vi "WildDrive_v4.vi"(8 "Defense Mode":bool, 9 "Enter Pivot":bool, 10 "Turn Joystick":dbl, 11 "Speed Joystick":dbl=-0.0) -> (0 "Right Side Power":dbl, 3 "Left Side Power":dbl)   [LabVIEW 2018]
uses:
  <vilib>/Analysis/1siggen.llb/Ramp Pattern by Samples.vi
  <vilib>/Analysis/NI_AALBase.lvlib
panel:
  in  "Debug Mode":bool
  in  "Debug Speed":dbl(slide) min=-1.0 max=1.0 scale=-1.0..1.0
  in  "Square Speed":bool=TRUE
  in  "Feed Forward Coeff":dbl(slide)=0.05 min=0.0 max=0.2 scale=0.0..0.2
  in  "Max Pivot Turn (defense)":dbl(slide)=0.05 min=0.0 max=1.0 scale=0.0..1.0
  in  "Max Pivot Turn (offense)":dbl(slide)=0.05 min=0.0 max=1.0 scale=0.0..1.0
  in  "Tune Arc Turn":dbl(slide)=1.2 min=0.9 max=2.0 scale=0.9..2.0
  in  "Speed Joystick Deadband":dbl(slide)=0.05 min=0.0 max=1.0 scale=0.0..1.0
  in  "Turn Behavior":bool=TRUE
  out "Left Side Power":cluster{"Y":dbl[], "X":dbl[]}(graph)={"Y"=[0.0, 0.010101010101010102, 0.020202020202020204, 0.030303030303030304, 0.04040404040404041, 0.05050505050505051, 0.06060606060606061, 0.07070707070707072, 0.08080808080808081, 0.09090909090909091, 0.10101010101010102, 0.11111111111111112, 0.12121212121212122, 0.13131313131313133, 0.14141414141414144, 0.15151515151515152, 0.16161616161616163, 0.17171717171717174, 0.18181818181818182, 0.19191919191919193, 0.20202020202020204, 0.21212121212121213, 0.22222222222222224, 0.23232323232323235, 0.24242424242424243, 0.25252525252525254, 0.26262626262626265, 0.27272727272727276, 0.2828282828282829, 0.29292929292929293, 0.30303030303030304, 0.31313131313131315, 0.32323232323232326, 0.33333333333333337, 0.3434343434343435, 0.3535353535353536, 0.36363636363636365, 0.37373737373737376, 0.38383838383838387, 0.393939393939394, 0.4040404040404041, 0.4141414141414142, 0.42424242424242425, 0.43434343434343436, 0.4444444444444445, 0.4545454545454546, 0.4646464646464647, 0.4747474747474748, 0.48484848484848486, 0.494949494949495, 0.5050505050505051, 0.5151515151515152, 0.5252525252525253, 0.5353535353535354, 0.5454545454545455, 0.5555555555555556, 0.5656565656565657, 0.5757575757575758, 0.5858585858585859, 0.595959595959596, 0.6060606060606061, 0.6161616161616162, 0.6262626262626263, 0.6363636363636365, 0.6464646464646465, 0.6565656565656566, 0.6666666666666667, 0.6767676767676768, 0.686868686868687, 0.696969696969697, 0.7070707070707072, 0.7171717171717172, 0.7272727272727273, 0.7373737373737375, 0.7474747474747475, 0.7575757575757577, 0.7676767676767677, 0.7777777777777778, 0.787878787878788, 0.797979797979798, 0.8080808080808082, 0.8181818181818182, 0.8282828282828284, 0.8383838383838385, 0.8484848484848485, 0.8585858585858587, 0.8686868686868687, 0.8787878787878789, 0.888888888888889, 0.8989898989898991, 0.9090909090909092, 0.9191919191919192, 0.9292929292929294, 0.9393939393939394, 0.9494949494949496, 0.9595959595959597, 0.9696969696969697, 0.9797979797979799, 0.98989898989899, 1.0], "X"=[0.0]}
  out "Right Side Power":cluster{"Y":dbl[], "X":dbl[]}(graph)={"Y"=[0.0, 0.010101010101010102, 0.020202020202020204, 0.030303030303030304, 0.04040404040404041, 0.05050505050505051, 0.06060606060606061, 0.07070707070707072, 0.08080808080808081, 0.09090909090909091, 0.10101010101010102, 0.11111111111111112, 0.12121212121212122, 0.13131313131313133, 0.14141414141414144, 0.15151515151515152, 0.16161616161616163, 0.17171717171717174, 0.18181818181818182, 0.19191919191919193, 0.20202020202020204, 0.21212121212121213, 0.22222222222222224, 0.23232323232323235, 0.24242424242424243, 0.25252525252525254, 0.26262626262626265, 0.27272727272727276, 0.2828282828282829, 0.29292929292929293, 0.30303030303030304, 0.31313131313131315, 0.32323232323232326, 0.33333333333333337, 0.3434343434343435, 0.3535353535353536, 0.36363636363636365, 0.37373737373737376, 0.38383838383838387, 0.393939393939394, 0.4040404040404041, 0.4141414141414142, 0.42424242424242425, 0.43434343434343436, 0.4444444444444445, 0.4545454545454546, 0.4646464646464647, 0.4747474747474748, 0.48484848484848486, 0.494949494949495, 0.5050505050505051, 0.5151515151515152, 0.5252525252525253, 0.5353535353535354, 0.5454545454545455, 0.5555555555555556, 0.5656565656565657, 0.5757575757575758, 0.5858585858585859, 0.595959595959596, 0.6060606060606061, 0.6161616161616162, 0.6262626262626263, 0.6363636363636365, 0.6464646464646465, 0.6565656565656566, 0.6666666666666667, 0.6767676767676768, 0.686868686868687, 0.696969696969697, 0.7070707070707072, 0.7171717171717172, 0.7272727272727273, 0.7373737373737375, 0.7474747474747475, 0.7575757575757577, 0.7676767676767677, 0.7777777777777778, 0.787878787878788, 0.797979797979798, 0.8080808080808082, 0.8181818181818182, 0.8282828282828284, 0.8383838383838385, 0.8484848484848485, 0.8585858585858587, 0.8686868686868687, 0.8787878787878789, 0.888888888888889, 0.8989898989898991, 0.9090909090909092, 0.9191919191919192, 0.9292929292929294, 0.9393939393939394, 0.9494949494949496, 0.9595959595959597, 0.9696969696969697, 0.9797979797979799, 0.98989898989899, 1.0], "X"=[0.0]}
  in  "Turn Joystick Deadband":dbl(slide)=0.05 min=0.0 max=1.0 scale=0.0..1.0
  out "Speed Joystick Mapping":cluster{"Y":dbl[], "X":dbl[]}(graph)={"Y"=[0.0, 0.010101010101010102, 0.020202020202020204, 0.030303030303030304, 0.04040404040404041, 0.05050505050505051, 0.06060606060606061, 0.07070707070707072, 0.08080808080808081, 0.09090909090909091, 0.10101010101010102, 0.11111111111111112, 0.12121212121212122, 0.13131313131313133, 0.14141414141414144, 0.15151515151515152, 0.16161616161616163, 0.17171717171717174, 0.18181818181818182, 0.19191919191919193, 0.20202020202020204, 0.21212121212121213, 0.22222222222222224, 0.23232323232323235, 0.24242424242424243, 0.25252525252525254, 0.26262626262626265, 0.27272727272727276, 0.2828282828282829, 0.29292929292929293, 0.30303030303030304, 0.31313131313131315, 0.32323232323232326, 0.33333333333333337, 0.3434343434343435, 0.3535353535353536, 0.36363636363636365, 0.37373737373737376, 0.38383838383838387, 0.393939393939394, 0.4040404040404041, 0.4141414141414142, 0.42424242424242425, 0.43434343434343436, 0.4444444444444445, 0.4545454545454546, 0.4646464646464647, 0.4747474747474748, 0.48484848484848486, 0.494949494949495, 0.5050505050505051, 0.5151515151515152, 0.5252525252525253, 0.5353535353535354, 0.5454545454545455, 0.5555555555555556, 0.5656565656565657, 0.5757575757575758, 0.5858585858585859, 0.595959595959596, 0.6060606060606061, 0.6161616161616162, 0.6262626262626263, 0.6363636363636365, 0.6464646464646465, 0.6565656565656566, 0.6666666666666667, 0.6767676767676768, 0.686868686868687, 0.696969696969697, 0.7070707070707072, 0.7171717171717172, 0.7272727272727273, 0.7373737373737375, 0.7474747474747475, 0.7575757575757577, 0.7676767676767677, 0.7777777777777778, 0.787878787878788, 0.797979797979798, 0.8080808080808082, 0.8181818181818182, 0.8282828282828284, 0.8383838383838385, 0.8484848484848485, 0.8585858585858587, 0.8686868686868687, 0.8787878787878789, 0.888888888888889, 0.8989898989898991, 0.9090909090909092, 0.9191919191919192, 0.9292929292929294, 0.9393939393939394, 0.9494949494949496, 0.9595959595959597, 0.9696969696969697, 0.9797979797979799, 0.98989898989899, 1.0], "X"=[0.0]}
  out "Turn Joystick Mapping":cluster{"Y":dbl[], "X":dbl[]}(graph)={"Y"=[0.0, 0.010101010101010102, 0.020202020202020204, 0.030303030303030304, 0.04040404040404041, 0.05050505050505051, 0.06060606060606061, 0.07070707070707072, 0.08080808080808081, 0.09090909090909091, 0.10101010101010102, 0.11111111111111112, 0.12121212121212122, 0.13131313131313133, 0.14141414141414144, 0.15151515151515152, 0.16161616161616163, 0.17171717171717174, 0.18181818181818182, 0.19191919191919193, 0.20202020202020204, 0.21212121212121213, 0.22222222222222224, 0.23232323232323235, 0.24242424242424243, 0.25252525252525254, 0.26262626262626265, 0.27272727272727276, 0.2828282828282829, 0.29292929292929293, 0.30303030303030304, 0.31313131313131315, 0.32323232323232326, 0.33333333333333337, 0.3434343434343435, 0.3535353535353536, 0.36363636363636365, 0.37373737373737376, 0.38383838383838387, 0.393939393939394, 0.4040404040404041, 0.4141414141414142, 0.42424242424242425, 0.43434343434343436, 0.4444444444444445, 0.4545454545454546, 0.4646464646464647, 0.4747474747474748, 0.48484848484848486, 0.494949494949495, 0.5050505050505051, 0.5151515151515152, 0.5252525252525253, 0.5353535353535354, 0.5454545454545455, 0.5555555555555556, 0.5656565656565657, 0.5757575757575758, 0.5858585858585859, 0.595959595959596, 0.6060606060606061, 0.6161616161616162, 0.6262626262626263, 0.6363636363636365, 0.6464646464646465, 0.6565656565656566, 0.6666666666666667, 0.6767676767676768, 0.686868686868687, 0.696969696969697, 0.7070707070707072, 0.7171717171717172, 0.7272727272727273, 0.7373737373737375, 0.7474747474747475, 0.7575757575757577, 0.7676767676767677, 0.7777777777777778, 0.787878787878788, 0.797979797979798, 0.8080808080808082, 0.8181818181818182, 0.8282828282828284, 0.8383838383838385, 0.8484848484848485, 0.8585858585858587, 0.8686868686868687, 0.8787878787878789, 0.888888888888889, 0.8989898989898991, 0.9090909090909092, 0.9191919191919192, 0.9292929292929294, 0.9393939393939394, 0.9494949494949496, 0.9595959595959597, 0.9696969696969697, 0.9797979797979799, 0.98989898989899, 1.0], "X"=[-0.0]}
  # "Driver Inputs"
  # "Tuning Parameters"
  # "Debug"
  # "Drive Outputs"
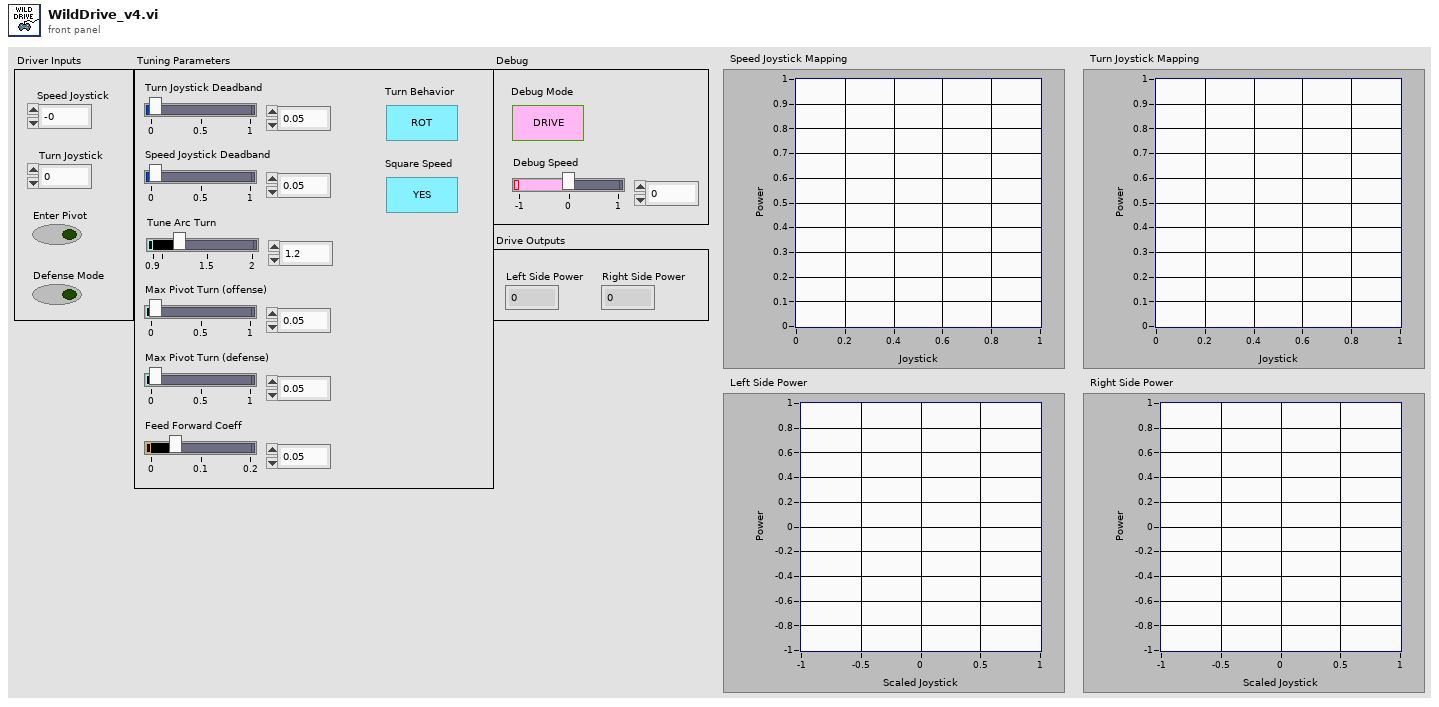
[diagram p1: front panel]
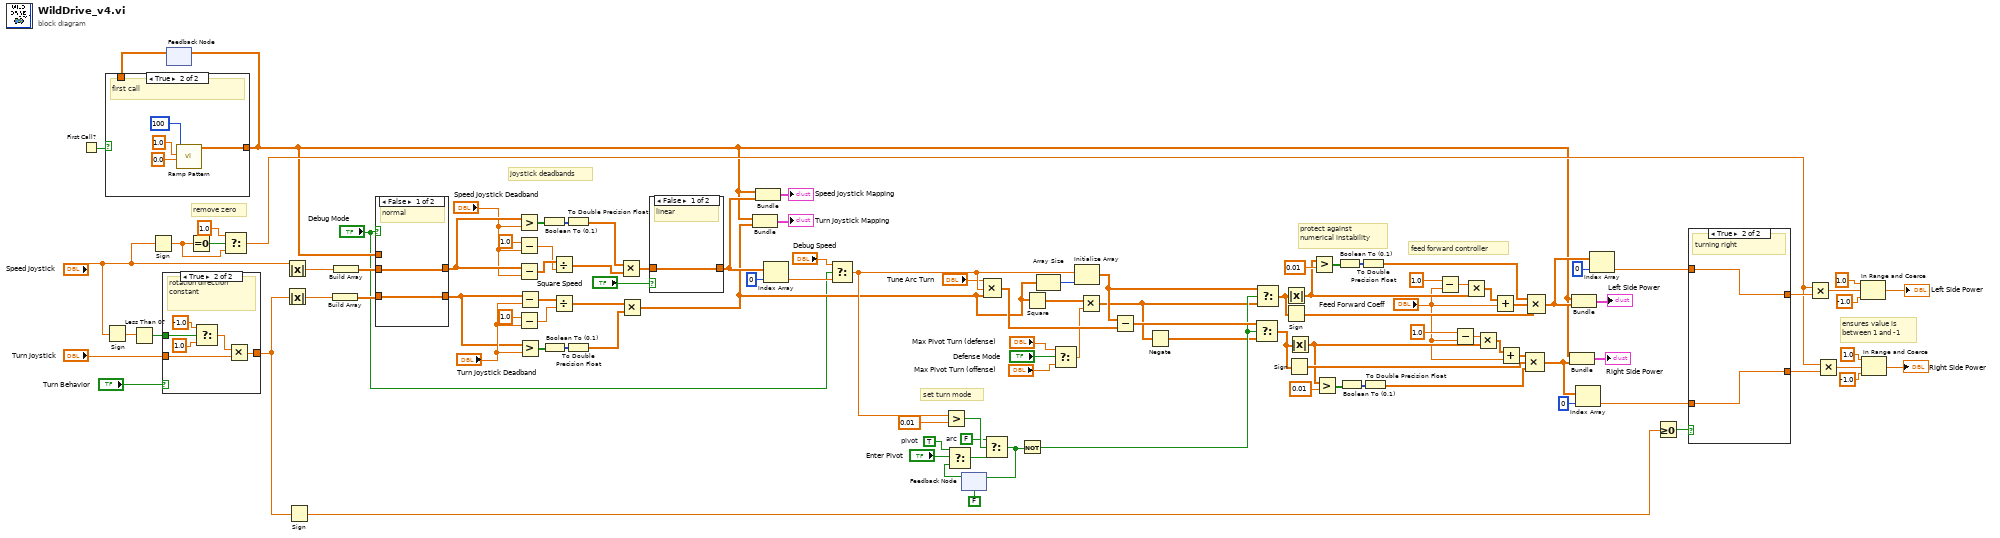
[diagram p0: block diagram]
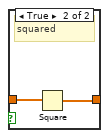
[diagram p6: hidden frame]
diagram:
  w12 = TRUE  # pivot
  w72 = FALSE  # arc
  # "remove zero"
  # "protect against\nnumerical instability"
  # "ensures value is \nbetween 1 and -1"
  # "set turn mode"
  # "feed forward controller"
  # "joystick deadbands"
  n1 = First Call?() -> (First Call?: T/F=w15:bool)
  n2 = Sign(1:"Speed Joystick") -> (0:w26:dbl)
  n3 = Less Than 0?(x=w26) -> (x < 0?=w27:bool)
  n4 = Sign(1:"Speed Joystick") -> (0:w19:dbl)
  n5 = case shown="True" "Turn Behavior" {
    tunnel: w27 -> [_ w117]
    tunnel: [w112 w114] -> w22
    tunnel: "Turn Joystick" -> [w112 w113]
    frame False {
      # "like a car"
    }
    frame True {
      # "rotation direction constant"
      n6 = Select(t=-1.0, s=w117, f=1.0) -> (s? t:f=w118:dbl)
      n7 = Multiply(x=w118, y=w113) -> (x*y=w114:dbl)
    }
  }
  n8 = feedback #1() -> (w13:dbl[])  [unwired: 1 in]
  n9 = case shown="True" w15 {
    tunnel: [w119 w120] -> w14
    tunnel: w13 -> [w119 _]
    frame False {
      # "subsequent calls"
    }
    frame True {
      # "first call"
      n10 = call-poly <vilib>:"Ramp Pattern.vi"("start"=0.0, "end"=1.0, "samples"=100) -> ("Ramp Pattern"=w120:dbl[])  [unwired: 7 in, 1 out]
    }
  }
  n11 = feedback-in #1(w14) -> ()
  n12 = Equal To 0?(x=w19) -> (x = 0?=w21:bool)
  n13 = Select(t=1.0, s=w21, f=w19) -> (s? t:f=w18:dbl)
  n14 = Absolute Value(x="Speed Joystick") -> (abs(x)=w108:dbl)
  n15 = Absolute Value(x=w22) -> (abs(x)=w111:dbl)
  n16 = Sign(1:w22) -> (0:w32:dbl)
  n17 = Build Array(w111) -> (w109:dbl[])
  n18 = Build Array(w108) -> (w110:dbl[])
  n19 = case shown="False" "Debug Mode" {
    tunnel: w14 -> [_ w126]
    tunnel: [w125 w126] -> w99
    tunnel: [w124 w126] -> w90
    tunnel: w110 -> [w125 _]
    tunnel: w109 -> [w124 _]
    frame False {
      # "normal"
    }
    frame True {
      # "debug"
    }
  }
  n20 = Greater?(x=w99, y="Speed Joystick Deadband") -> (0:w105:bool[])
  n21 = Subtract(x=1.0, y="Speed Joystick Deadband") -> (x-y=w96:dbl)
  n22 = Subtract(x=w99, y="Speed Joystick Deadband") -> (x-y=w98:dbl[])
  n23 = Subtract(x=1.0, y="Turn Joystick Deadband") -> (x-y=w92:dbl)
  n24 = Subtract(x=w90, y="Turn Joystick Deadband") -> (x-y=w94:dbl[])
  n25 = Greater?(x=w90, y="Turn Joystick Deadband") -> (0:w103:bool[])
  n26 = Boolean To (0,1)(Boolean=w105) -> (0, 1=w104:i16[])
  n27 = Boolean To (0,1)(Boolean=w103) -> (0, 1=w102:i16[])
  n28 = Divide(x=w98, y=w96) -> (x/y=w95:dbl[])
  n29 = Divide(x=w94, y=w92) -> (x/y=w89:dbl[])
  n30 = To Double Precision Float(number=w104) -> (double precision float=w101:dbl[])
  n31 = To Double Precision Float(number=w102) -> (double precision float=w88:dbl[])
  n32 = Multiply(x=w101, y=w95) -> (x*y=w100:dbl[])
  n33 = Multiply(x=w89, y=w88) -> (x*y=w3:dbl[])
  n34 = case shown="False" "Square Speed" {
    tunnel: w100 -> [w127 w129]
    tunnel: [w127 w128] -> w76
    frame False {
      # "linear"
    }
    frame True {
      # "squared"
      n35 = Square(x=w129) -> (x^2=w128:dbl[])
    }
  }
  n36 = Bundle("Ramp Pattern"=w14, w3) -> (→"Turn Joystick Mapping":cluster{"Ramp Pattern":dbl[], dbl[]})  [unwired: 1 in]
  n37 = Bundle("Ramp Pattern"=w14, w76) -> (→"Speed Joystick Mapping":cluster{"Ramp Pattern":dbl[], dbl[]})  [unwired: 1 in]
  n38 = Index Array(array=w76, index=0) -> (element=w78:dbl)
  n39 = Select(t="Debug Speed", s="Debug Mode", f=w78) -> (s? t:f=w31:dbl)
  n40 = Greater?(x=w31, y=0.01) -> (0:w74:bool)
  n41 = feedback #2(FALSE) -> (w80:bool)
  n42 = Select(t=w12, s="Enter Pivot", f=w80) -> (s? t:f=w73:bool)
  n43 = Compound Arithmetic op=MULTIPLY("Tune Arc Turn", w31, w3) -> (w82:dbl[])
  n44 = Select(t=w72, s=w74, f=w73) -> (s? t:f=w71:bool)
  n45 = feedback-in #2(w71) -> ()
  n46 = Not(x=w71) -> (.not. x?=w70:bool)
  n47 = Square(x=w3) -> (x^2=w17:dbl[])
  n48 = Array Size(array=w3) -> (size(s)=w87:i32)
  n49 = Select(t="Max Pivot Turn (defense)", s="Defense Mode", f="Max Pivot Turn (offense)") -> (s? t:f=w11:dbl)
  n50 = Initialize Array(w31, w87) -> (w86:dbl[])
  n51 = Multiply(x=w17, y=w11) -> (x*y=w16:dbl[])
  n52 = Subtract(x=w86, y=w82) -> (x-y=w85:dbl[])
  n53 = Negate(x=w16) -> (-x=w69:dbl[])
  n54 = Select(t=w85, s=w70, f=w69) -> (s? t:f=w30:dbl[])
  n55 = Select(t=w86, s=w70, f=w16) -> (s? t:f=w52:dbl[])
  n56 = Sign(1:w52) -> (0:w65:dbl[])
  n57 = Absolute Value(x=w52) -> (abs(x)=w28:dbl[])
  n58 = Sign(1:w30) -> (0:w60:dbl[])
  n59 = Absolute Value(x=w30) -> (abs(x)=w29:dbl[])
  n60 = Greater?(x=w28, y=0.01) -> (0:w55:bool[])
  n61 = Greater?(x=w29, y=0.01) -> (0:w59:bool[])
  n62 = Boolean To (0,1)(Boolean=w55) -> (0, 1=w54:i16[])
  n63 = Boolean To (0,1)(Boolean=w59) -> (0, 1=w58:i16[])
  n64 = To Double Precision Float(number=w54) -> (double precision float=w51:dbl[])
  n65 = To Double Precision Float(number=w58) -> (double precision float=w56:dbl[])
  n66 = Subtract(x=1.0, y="Feed Forward Coeff") -> (x-y=w67:dbl)
  n67 = Subtract(x=1.0, y="Feed Forward Coeff") -> (x-y=w63:dbl)
  n68 = Multiply(x=w67, y=w28) -> (x*y=w66:dbl[])
  n69 = Multiply(x=w63, y=w29) -> (x*y=w62:dbl[])
  n70 = Add(x=w66, y="Feed Forward Coeff") -> (x+y=w50:dbl[])
  n71 = Add(x=w62, y="Feed Forward Coeff") -> (x+y=w61:dbl[])
  n72 = Compound Arithmetic op=MULTIPLY(w61, w60, w56) -> (w48:dbl[])
  n73 = Compound Arithmetic op=MULTIPLY(w51, w50, w65) -> (w46:dbl[])
  n74 = Bundle("Ramp Pattern"=w14, w48) -> (→"Right Side Power":cluster{"Ramp Pattern":dbl[], dbl[]})  [unwired: 1 in]
  n75 = Bundle("Ramp Pattern"=w14, w46) -> (→"Left Side Power":cluster{"Ramp Pattern":dbl[], dbl[]})  [unwired: 1 in]
  n76 = Index Array(array=w48, index=0) -> (element=w35:dbl)
  n77 = Index Array(array=w46, index=0) -> (element=w37:dbl)
  n78 = Greater Or Equal To 0?(x=w32) -> (x >= 0?=w33:bool)
  n79 = case shown="True" w33 {
    tunnel: w37 -> [w131 w133]
    tunnel: [w130 w133] -> w36
    tunnel: w35 -> [w130 w132]
    tunnel: [w131 w132] -> w34
    frame False {
      # "turning left"
    }
    frame True {
      # "turning right"
    }
  }
  n80 = Multiply(x=w18, y=w36) -> (x*y=w38:dbl)
  n81 = Multiply(x=w18, y=w34) -> (x*y=w39:dbl)
  n82 = In Range and Coerce(upper limit=1.0, x=w38, lower limit=-1.0) -> (coerced(x)=→"Left Side Power":dbl)  [unwired: 1 out]
  n83 = In Range and Coerce(upper limit=1.0, x=w39, lower limit=-1.0) -> (coerced(x)=→"Right Side Power":dbl)  [unwired: 1 out]
